vi "DSF.Engine.Transfer.Set Configuration.vi"(10 "Configuration":refnum<class "DSF.Shared.Configuration.Transfer.lvclass">, 11 "Transfer in":refnum<class "DSF.Engine.Transfer.lvclass">) -> (3 "Transfer out":refnum<class "DSF.Engine.Transfer.lvclass">)   [LabVIEW 2016, in "DSF.Engine.lvlib" / "DSF.Engine.Transfer.lvclass"]
uses:
  DSF.Engine.Transfer.lvclass
  Shared/Classes/Transfer/DSF.Shared.Configuration.Transfer.lvclass
  DSF.Engine.Transfer.lvclass/DSF.Engine.Transfer.ctl
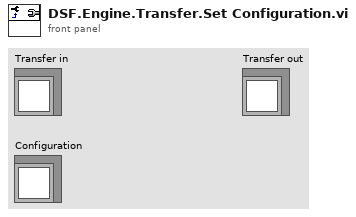
[diagram p1: front panel]
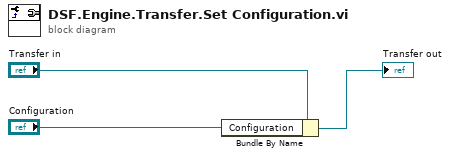
[diagram p0: block diagram]
diagram:
  n1 = Bundle By Name(cluster="Transfer in", "Configuration"="Configuration") -> (→"Transfer out":refnum<class "DSF.Engine.Transfer.lvclass">)
